vi "Append to Content.vi"(8 "error in (no error)":errorcluster {"code" format="Error %.0f"}, 10 "Content":string, 11 "VIDoc Printer - Confluence In":refnum<class "VIDoc Printer - Confluence.lvclass">) -> (0 "error out":errorcluster {"code" format="Error %.0f"}, 3 "VIDoc Printer - Confluence Out":refnum<class "VIDoc Printer - Confluence.lvclass">)   [LabVIEW 2023, in "VIDoc Printer - Confluence.lvlib" / "VIDoc Printer - Confluence.lvclass"]
uses:
  VIDoc Printer - Confluence.lvclass
  VIDoc Printer - Confluence.lvclass/VIDoc Printer - Confluence.ctl
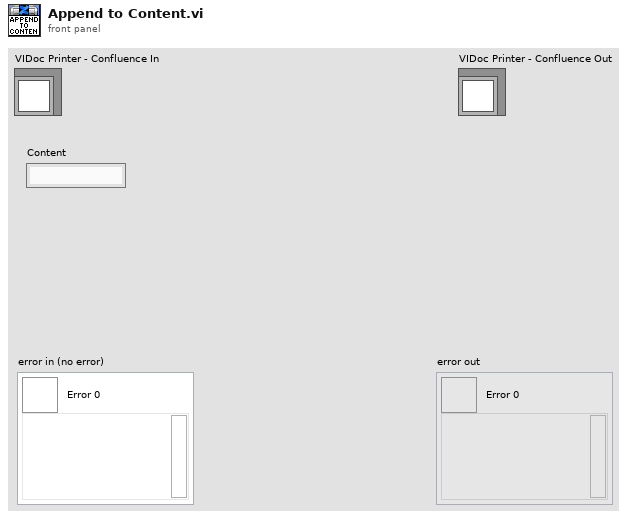
[diagram p1: front panel]
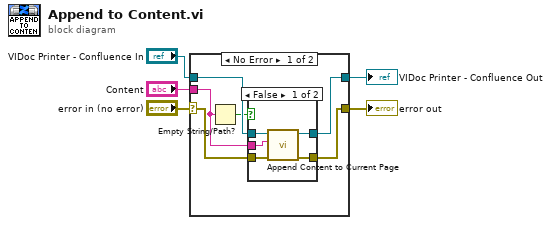
[diagram p0: block diagram]
diagram:
  n1 = case shown="No Error" "error in (no error)" {
    selector: "error in (no error)" -> [w9 w20]
    tunnel: [w8 w20] -> w4
    tunnel: [w10 w19] -> w2
    tunnel: "VIDoc Printer - Confluence In" -> [w11 w19]
    tunnel: "Content" -> [w6 _]
    frame No Error {
      n2 = Empty String/Path?(string/path=w6) -> (empty?=w7:bool)
      n3 = case shown="False" w7 {
        tunnel: w11 -> [w16 w17]
        tunnel: [w15 w17] -> w10
        tunnel: w9 -> [w14 w18]
        tunnel: [w13 w18] -> w8
        tunnel: w6 -> [w12 _]
        frame False {
          n4 = call "Append Content to Current Page.vi"("error in (no error)"=w14, "Content"=w12, "Conf Printer in"=w16) -> ("error out"=w13:errorcluster, "Conf Printer out"=w15:refnum<class "VIDoc Printer - Confluence.lvclass">)  [unwired: 7 in]
        }
        frame True {
        }
      }
    }
    frame Error {
    }
  }
  "error out" <- w4
  "VIDoc Printer - Confluence Out" <- w2
